vi "Run_Core.vi"(0 "Booelan Operations in":refnum<class "Boolean Functions.lvclass">, 11 "error in (no error)":errorcluster) -> (4 "Booelan Operations out":refnum<class "Boolean Functions.lvclass">, 6 "Return":variant, 15 "error out":errorcluster)   [LabVIEW 2019, in "Boolean Functions.lvclass"]
uses:
  Boolean Functions.lvclass
  Boolean Functions.lvclass/Boolean Functions.ctl
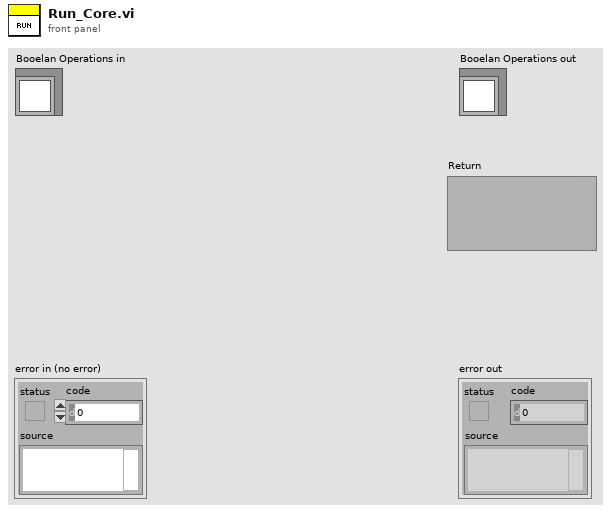
[diagram p1: front panel]
types:
  T1 = typedef "Boolean Functions.lvclass/Function List.ctl" = enum16{"And", "Or", "Exclusive Or", "Not", "Not And", "Not Or", "Not Exclusive Or", "Random Bool"}
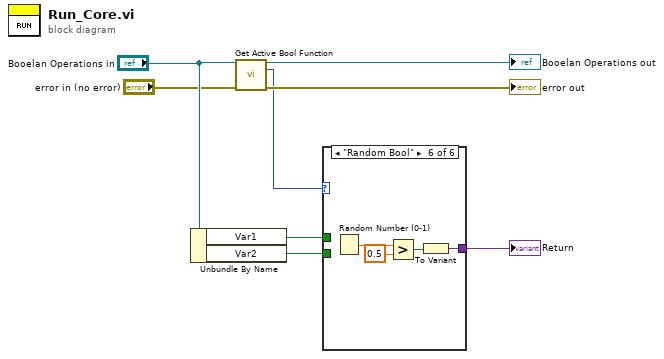
[diagram p0: block diagram]
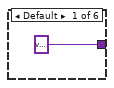
[diagram p2: hidden frame]
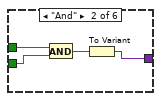
[diagram p3: hidden frame]
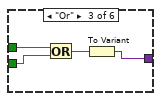
[diagram p4: hidden frame]
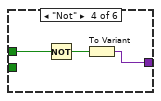
[diagram p5: hidden frame]
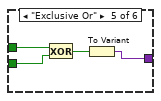
[diagram p6: hidden frame]
diagram:
  n1 = Unbundle By Name("Booelan Operations in") -> ("Var1"=w8:bool, "Var2"=w7:bool)
  n2 = call "Get Active Bool Function.vi"("Boolean Functions in"="Booelan Operations in", "error in (no error)"="error in (no error)") -> ("Boolean Functions out"=→"Booelan Operations out":refnum<class "Boolean Functions.lvclass">, "Function"=w1:T1, "error out"=→"error out":errorcluster)  [unwired: 11 in]
  n3 = case shown="\"Random Bool\"" w1 {
    tunnel: w8 -> [_ w13 w17 w20 w24 _]
    tunnel: w7 -> [_ w12 w16 _ w23 _]
    tunnel: [variant ("Variant") w10 w14 w18 w21 w25] -> w6
    frame Default {
    }
    frame "And" {
      n4 = And(x=w13, y=w12) -> (x .and. y?=w11:bool)
      n5 = To Variant(anything=w11) -> (Variant=w10:variant)
    }
    frame "Or" {
      n6 = Or(x=w17, y=w16) -> (x .or. y?=w15:bool)
      n7 = To Variant(anything=w15) -> (Variant=w14:variant)
    }
    frame "Not" {
      n8 = Not(x=w20) -> (.not. x?=w19:bool)
      n9 = To Variant(anything=w19) -> (Variant=w18:variant)
    }
    frame "Exclusive Or" {
      n10 = Exclusive Or(1:w23, 2:w24) -> (0:w22:bool)
      n11 = To Variant(anything=w22) -> (Variant=w21:variant)
    }
    frame "Random Bool" {
      n12 = Random Number (0-1)() -> (number: 0 to 1=w28:dbl)
      n13 = Greater?(x=w28, y=0.5) -> (0:w26:bool)
      n14 = To Variant(anything=w26) -> (Variant=w25:variant)
    }
  }
  "Return" <- w6
